vi "gespielte leider.vi"(1 "Referenz 3":refnum<vi>, 2 "Referenz 2":refnum<vi>, 3 "Referenz":refnum<vi>) -> ()   [LabVIEW 2010]
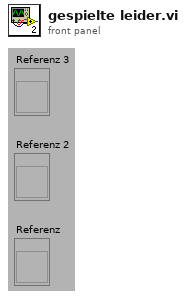
[diagram p1: front panel]
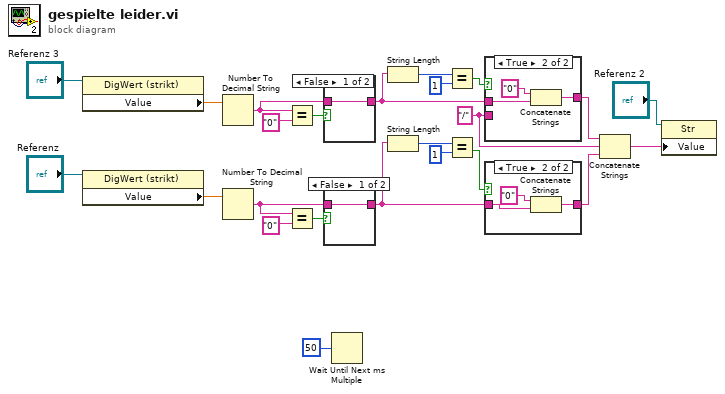
[diagram p0: block diagram]
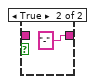
[diagram p2: hidden frame]
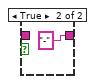
[diagram p3: hidden frame]
diagram:
  w8 = "/"
  n1 = property class="DigWert (strikt)"(reference="Referenz 3") -> ("Value"=w16:dbl)  [unwired: 1 in, 2 out]
  n2 = property class="DigWert (strikt)"(reference="Referenz") -> ("Value"=w13:dbl)  [unwired: 1 in, 2 out]
  n3 = Number To Decimal String(number=w16) -> (decimal integer string=w24:string)  [unwired: 1 out]
  n4 = Number To Decimal String(number=w13) -> (decimal integer string=w20:string)  [unwired: 1 out]
  n5 = Equal?(x=w24, y="0") -> (x = y?=w22:bool)
  n6 = Equal?(x=w20, y="0") -> (x = y?=w18:bool)
  n7 = case shown="FALSE" w22 {
    tunnel: [w25 "-"] -> w23
    tunnel: w24 -> [w25 _]
    frame False {
    }
    frame True {
    }
  }
  n8 = case shown="FALSE" w18 {
    tunnel: [w27 "-"] -> w19
    tunnel: w20 -> [w27 _]
    frame False {
    }
    frame True {
    }
  }
  n9 = Wait Until Next ms Multiple(millisecond multiple=50) -> ()  [unwired: 1 out]
  n10 = String Length(string=w23) -> (length=w5:i32)
  n11 = String Length(string=w19) -> (length=w10:i32)
  n12 = Equal?(x=w5, y=1) -> (x = y?=w7:bool)
  n13 = Equal?(x=w10, y=1) -> (x = y?=w12:bool)
  n14 = case shown="TRUE" w7 {
    tunnel: w23 -> [w29 w31]
    tunnel: w8 -> [_ _]
    tunnel: [w29 w30] -> w9
    frame False {
    }
    frame True {
      n15 = Concatenate Strings("0" ("String"), w31) -> (w30:string)
    }
  }
  n16 = case shown="TRUE" w12 {
    tunnel: w19 -> [w33 w35]
    tunnel: [w33 w34] -> w14
    frame False {
    }
    frame True {
      n17 = Concatenate Strings("0" ("String"), w35) -> (w34:string)
    }
  }
  n18 = Concatenate Strings(w9, w8, w14) -> (w15:string)
  n19 = property class="Str"(reference="Referenz 2", "Value"=w15) -> ()  [unwired: 1 in, 2 out]
